vi "ParseStringTo1Darray.vi"(11 "Copied Input From Advent Of Code Website":string) -> (3 "Formatted 1D String Array":string[](array[string]))   [LabVIEW 2021]
doc: "Parses source string into 1D String Array"
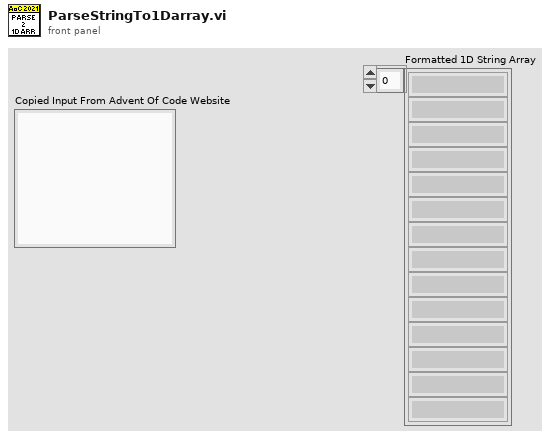
[diagram p1: front panel]
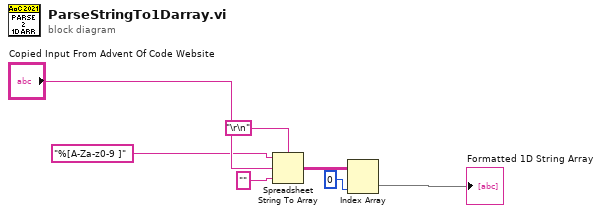
[diagram p0: block diagram]
diagram:
  n1 = Spreadsheet String To Array(delimiter (Tab)="\r\n", format string="%[A-Za-z0-9 ]", spreadsheet string="Copied Input From Advent Of Code Website", array type (2D Dbl)="" ("string")) -> (array=w3:string[][])
  n2 = Index Array(array=w3, index (col)=0 ("disabled index (col)")) -> (element=→"Formatted 1D String Array":string[])  [unwired: 1 in]
